vi "Serial FGV.vi"(6 "delay before read (ms)":u32=100, 7 "Status":enum16{"Config", "Read", "Write", "Close"}(ring), 8 "Error In":errorcluster={"status"=FALSE, "code"=1073676294, "source"="VISA Read in Serial Read.vi->Serial FGV.vi->Cascade Compressor Inverter.vi"}, 9 "Command":string="*IDN?", 10 "Serial Settings":T1={"baud rate"=19200, "data bits"=8, "parity"=enum."None", "stop bits"=10, "flow control"=0} {"flow control" items=["None"=0, "XON/XOFF"=1, "RTS/CTS"=2, "DTR/DSR"=4]; "stop bits" items=["1.0"=10, "1.5"=15, "2.0"=20]; "data bits" min=5 max=8 step=1; "baud rate" items=["75"=75, "110"=110, "134"=134, "150"=150, "300"=300, "600"=600, "1200"=1200, "1800"=1800, "2400"=2400, "4800"=4800, "7200"=7200, "9600"=9600, "14400"=14400, "19200"=19200, "28800"=28800, "38400"=38400, "56000"=56000, "57600"=57600, "115200"=115200, "128000"=128000, "230400"=230400]}, 11 "VISA resource name":refnum<visa-resource-name>="COM5") -> (0 "Error Out":errorcluster={"status"=TRUE, "code"=-1073807343, "source"="Property Node (arg 1) in VISA Configure Serial Port (Instr).vi->RS232 FGV.vi"}, 1 "return count":u32, 2 "bytes read":u32, 3 "Response":string)   [LabVIEW 2019, in "GUI.lvlib"]
uses:
  <vilib>/Instr/_visa.llb/VISA Configure Serial Port (Instr).vi
  GUI.lvlib
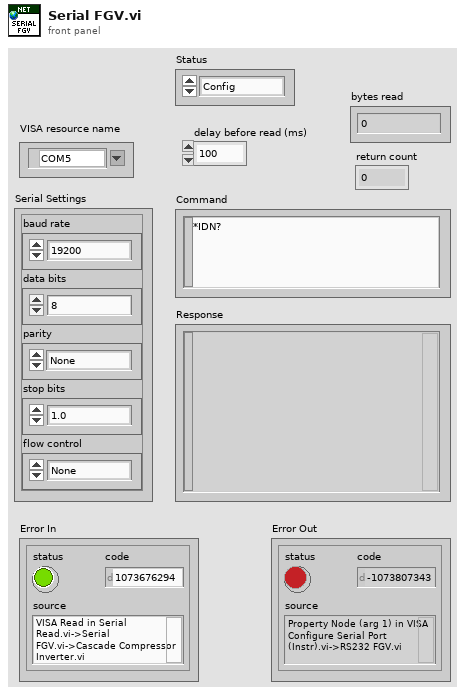
[diagram p1: front panel]
types:
  T1 = cluster{"baud rate":u32, "data bits":u16, "parity":enum16{"None", "Odd", "Even", "Mark", "Space"}, "stop bits":u16, "flow control":u16}
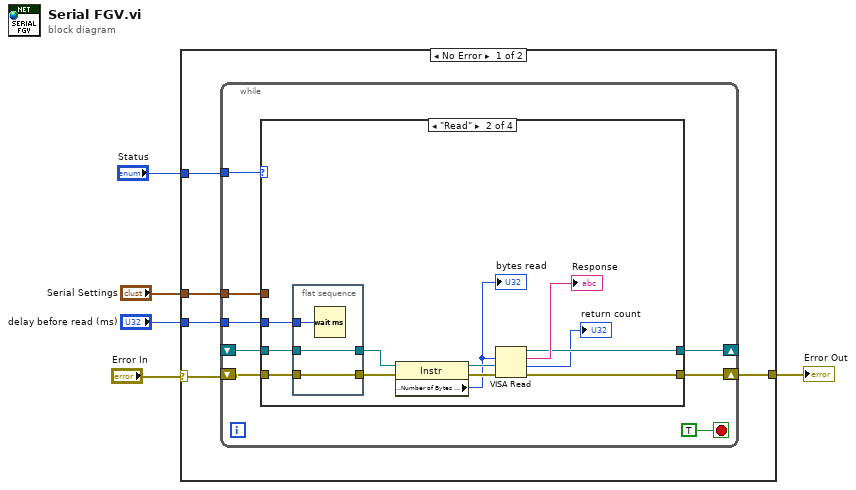
[diagram p0: block diagram]
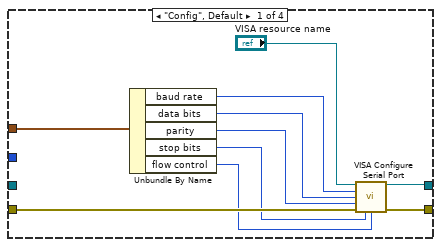
[diagram p2: hidden frame]
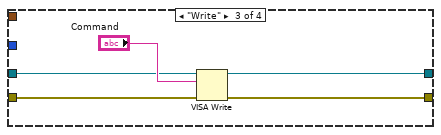
[diagram p3: hidden frame]
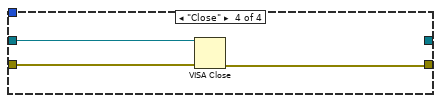
[diagram p4: hidden frame]
diagram:
  n1 = case shown="No Error" "Error In" {
    selector: "Error In" -> [w10 w52]
    tunnel: [w9 w52] -> w4
    tunnel: "delay before read (ms)" -> [w8 _]
    tunnel: "Serial Settings" -> [w7 _]
    tunnel: "Status" -> [w6 _]
    frame No Error {
      n2 = while {
        tunnel: w6 -> [w17]
        shift-right: [w16] -> w9
        shift-left: w10 -> [w15]
        shift-right: [w14] -> _
        shift-left: _ -> [w13]
        tunnel: w7 -> [w12]
        tunnel: w8 -> [w11]
        stop <- TRUE stop-if-true
        n3 = case shown="\"Read\"" w17 {
          tunnel: [w26 w37 w47 w50] -> w16
          tunnel: w15 -> [w27 w40 w48 w51]
          tunnel: [w20 w35 w44 _] -> w14
          tunnel: w13 -> [_ w39 w45 w49]
          tunnel: w12 -> [w19 _ _ _]
          tunnel: w11 -> [_ w38 _ _]
          frame "Config", Default {
            n4 = Unbundle By Name(w19) -> ("baud rate"=w25:u32, "data bits"=w24:u16, "parity"=w23:enum16{"None", "Odd", "Even", "Mark", "Space"}, "stop bits"=w22:u16, "flow control"=w21:u16)
            n5 = call-poly "VISA Configure Serial Port"("VISA resource name"="VISA resource name", "baud rate (9600)"=w25, "data bits (8)"=w24, "parity (0:none)"=w23, "error in (no error)"=w27, "stop bits (10: 1 bit)"=w22, "flow control (0:none)"=w21) -> ("VISA resource name out"=w20:refnum<visa-resource-name>, "error out"=w26:errorcluster)  [unwired: 3 in, 4 out]
          }
          frame "Read" {
            n6 = flat-sequence {
              tunnel: w40 -> [w43]
              tunnel: [w43] -> w34
              tunnel: w39 -> [w42]
              tunnel: [w42] -> w33
              tunnel: w38 -> [w41]
              frame #0 {
                n7 = Wait (ms)(milliseconds to wait=w41) -> ()  [unwired: 1 out]
              }
            }
            n8 = property class="Instr"(reference=w33, error in=w34) -> (reference out=w32:refnum<visa-resource-name>, error out=w31:errorcluster, "Serial Settings:Number of Bytes at Serial Port"=w30:u32)
            "bytes read" <- w30
            n9 = VISA Read(VISA resource name=w32, byte count=w30, error in (no error)=w31) -> (VISA resource name out=w35:refnum<visa-resource-name>, read buffer=→"Response":string, return count=→"return count":u32, error out=w37:errorcluster)
          }
          frame "Write" {
            n10 = VISA Write(VISA resource name=w45, write buffer="Command", error in (no error)=w48) -> (VISA resource name out=w44:refnum<visa-resource-name>, error out=w47:errorcluster)  [unwired: 1 out]
          }
          frame "Close" {
            n11 = VISA Close(VISA resource name=w49, error in (no error)=w51) -> (error out=w50:errorcluster)
          }
        }
      }
    }
    frame Error {
    }
  }
  "Error Out" <- w4
